vi "Get RSSI.vi"(10 "BLE Server Name":string, 11 "CMD Monitor":string="\r\n\n__STATUS__\r\nSTAUS: Idle\r\n\n__CONNECT__\r\n=> BLE-Device found: Name: , Address: 02:9e:20:bf:38:c3, manufacturer data: 0600010f2002ac4b9527554e76975feab6f01dfd2734f4a8d1b304ce2b, rssi: -90\r\n=> BLE-Device found: Name: , Address: 68:50:4d:fc:8d:fd, manufacturer data: 06000109200203d28ad0361826cc8c3442ea353b03bbfcafecf87a05fa, rssi: -46\r\n=> BLE-Device found: Name: , Address: 71:7c:fd:9e:68:f4, manufacturer data: 4c001006151abe80a526, txPower: 12, rssi: -79\r\n=> BLE-Device found: Name: , Address: 26:cf:d5:62:e8:21, manufacturer data: 060001092002071fdb04c7056e8d024be9531834bfd395421dc04640ed, rssi: -74\r\n=> BLE-Device found: Name: , Address: 1c:96:8d:3f:94:b6, manufacturer data: 0600010920028a9d70b2a55cf76c39f1e6c3aa216a18bc67a8bfa460a6, rssi: -79\r\n=> BLE-Device found: Name: , Address: 20:98:e7:43:ec:de, manufacturer data: 060001092002d7452958753618a94eddab88ed99627097bea80a0ee455, rssi: -91\r\n=> BLE-Device found: Name: , Address: 2d:79:9f:14:da:8a, manufacturer data: 060001092002ef0c23285ce8c8a4d9129dda5e8078c677fa5648740fa1, rssi: -65\r\n=> BLE-Device found: Name: , Address: 2f:f0:88:bb:aa:f4, manufacturer data: 060001092002847bff74a639f6fdbafe29abce9e42b2950e7085c963ea, rssi: -76\r\n=> BLE-Device found: Name: , Address: 5a:a3:29:bf:83:cd, manufacturer data: 4c00100523188deadc, txPower: 8, rssi: -82\r\n=> BLE-Device found: Name: , Address: 29:15:c1:95:c1:59, manufacturer data: 060001092002e10086f6f307213cb1f8aae23176b5c426ad22ca1f2735, rssi: -80\r\n=> BLE-Device found: Name: , Address: 0b:5b:c8:3f:71:c5, manufacturer data: 060001092002777e1dd530c0101c6e6af7e70c9fb392a21f029de9021a, rssi: -84\r\n=> BLE-Device found: Name: , Address: 4d:11:2d:15:bb:83, manufacturer data: 4c001006161eb5f9f4ff, txPower: 12, rssi: -87\r\n=> BLE-Device found: Name: , Address: 74:33:c9:81:a6:93, manufacturer data: 060001092002a1ad72a725548e7d17fa0e9a418d45822c03efced233e6, rssi: -86\r\n=> BLE-Device found: Name: , Address: 7c:b9:d9:dd:09:3e, manufacturer data: 060001092002173d877a61779ee2cdb22b360002842fb7f27ab856af47, rssi: -91\r\n=> BLE-Device found: Name: L21-1092, Address: 02:00:47:42:10:92, manufacturer data: 4a590200474210927b0028000800, serviceUUID: 0000fef5-0000-1000-8000-00805f9b34fb, serviceUUID: 00001812-0000-1000-8000-00805f9b34fb, rssi: -77\r\n=> BLE-Device found: Name: LEDLMS 2210070000001, Address: 6c:1d:eb:ad:8d:8a, serviceUUID: 2456e1b9-26e2-8f83-e744-f34f01e9d701, txPower: 4, rssi: -44\r\nForming a connection to 6c:1d:eb:ad:8d:8a\r\n=> Created client\r\n=> Connected to LMS-BLE server\r\n=> Found our service\r\n=> Found our characteristic\r\n=> Connected to LMS-BLE Server: PASS\r\n\n__LMS-CMD__\r\nopen\r\r\n\r\nChuck(3):> \n__LMS-CMD__\r\ngetPID\r\r\nPID: 2210070000001\r\n\r\nChuck(3):> \n__DISCONNECT__\r\n=> Diconnect from BLE-LMS Server.\r\n=>onDisconnect\r\n") -> (1 "rssi Str":string, 2 "rssi":i32, 3 "BLE LMS Server Found":bool)   [LabVIEW 2018]
panel:
  out "Array of Strings":string[](array[string])
  out "BLE Server Data":string
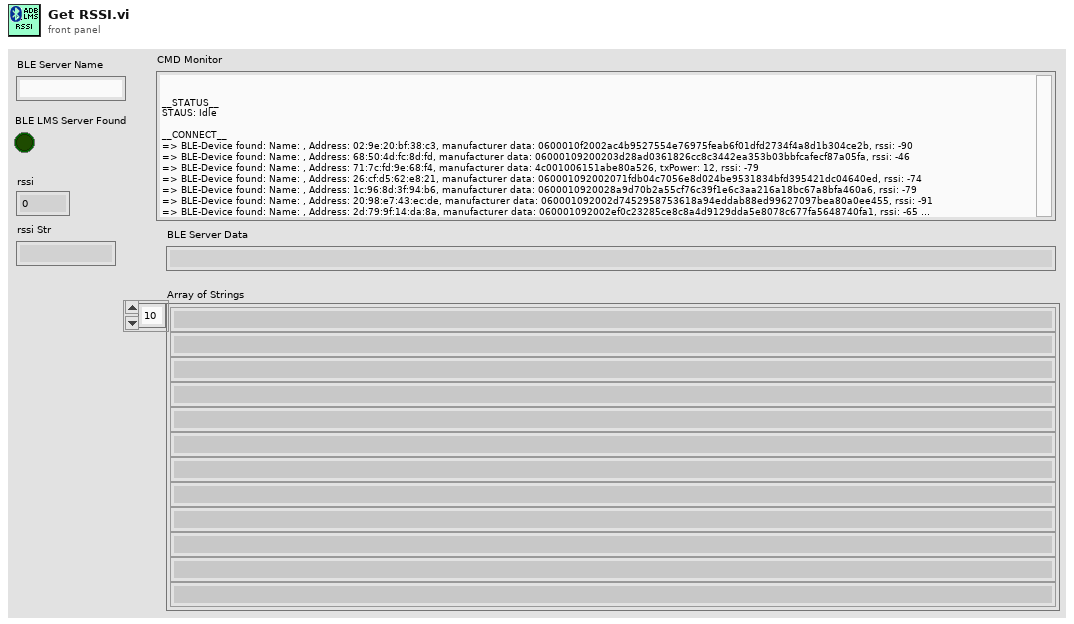
[diagram p1: front panel]
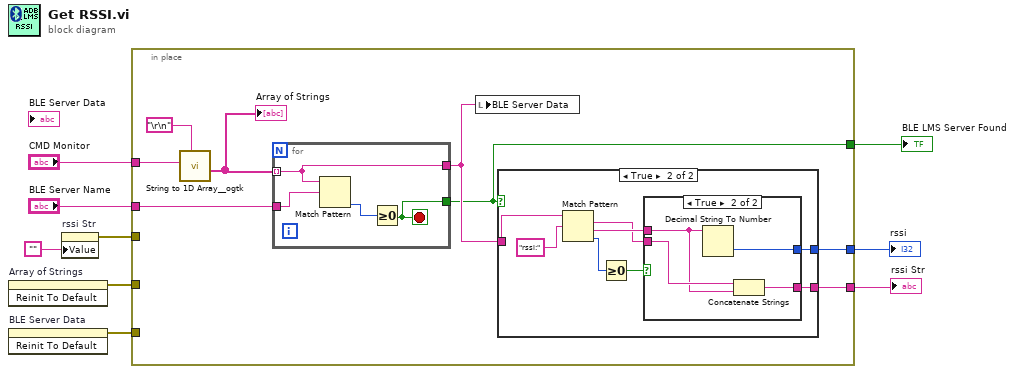
[diagram p0: block diagram]
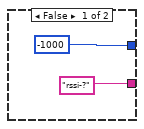
[diagram p2: hidden frame]
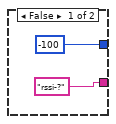
[diagram p3: hidden frame]
diagram:
  n1 = invoke on="Array of Strings" class="Arr (strict)" method="Reinit To Default"() -> (error out=w7:errorcluster)  [unwired: 3 in, 2 out]
  n2 = invoke on="BLE Server Data" class="Str" method="Reinit To Default"() -> (error out=w6:errorcluster)  [unwired: 3 in, 2 out]
  n3 = property on="rssi Str" class="Str"("Value"="") -> (error out=w2:errorcluster)  [unwired: 2 in, 1 out]
  n4 = in-place {
    in-place-border: "CMD Monitor" -> [w17]
    in-place-border: "BLE Server Name" -> [w14]
    in-place-border: w7 -> [_]
    in-place-border: w6 -> [_]
    in-place-border: [w12] -> w5
    in-place-border: [w11] -> w4
    in-place-border: [w10] -> w3
    in-place-border: w2 -> [_]
    n5 = call <userlib>:"String to 1D Array__ogtk.vi"("delimiter (Tab)"="\r\n", "string"=w17) -> ("Array of Strings"=w15:string[])  [unwired: 9 in]
    "Array of Strings" <- w15
    n6 = for {
      tunnel: w15 -> [w34] mode=indexing
      tunnel: w14 -> [w37]
      tunnel: [w34] -> w13
      tunnel: [w35] -> w11
      stop <- w35 stop-if-true
      n7 = Match Pattern(string=w34, regular expression=w37) -> (offset past match=w36:i32)  [unwired: 1 in, 3 out]
      n8 = Greater Or Equal To 0?(x=w36) -> (x >= 0?=w35:bool)
    }
    n9 = local write "BLE Server Data"(w13) -> ()
    n10 = case shown="True" w11 {
      tunnel: w13 -> [_ w27]
      tunnel: [-1000 w22] -> w12
      tunnel: ["rssi-?" w20] -> w10
      frame False {
      }
      frame True {
        n11 = Match Pattern(string=w27, regular expression="rssi:") -> (match substring=w21:string, after substring=w23:string, offset past match=w25:i32)  [unwired: 1 in, 1 out]
        n12 = Greater Or Equal To 0?(x=w25) -> (x >= 0?=w24:bool)
        n13 = case shown="True" w24 {
          tunnel: w23 -> [_ w30]
          tunnel: [-100 w33] -> w22
          tunnel: w21 -> [_ w32]
          tunnel: ["rssi-?" w31] -> w20
          frame False {
          }
          frame True {
            n14 = Decimal String To Number(string=w30) -> (number=w33:i32)  [unwired: 2 in, 1 out]
            n15 = Concatenate Strings(w32, w30) -> (w31:string)
          }
        }
      }
    }
  }
  "rssi" <- w5
  "BLE LMS Server Found" <- w4
  "rssi Str" <- w3
